vi "SE FP hindbrain ACT.vi"(4 "Manual?":bool=TRUE, 6 "error in":errorcluster, 7 "Act Com":T1, 8 "MHeading":dbl(slide) scale=-45.0..45.0 scale format="%_1f", 9 "MSpeed":dbl(slide) scale=-50.0..50.0 scale format="%#.1g") -> (0 "error out":errorcluster, 1 "Speed":dbl min=-9.0 max=9.0 step=1.0, 2 "Rudder":dbl min=-45.0 max=45.0 step=1.0, 3 "Desired\nSpeed":dbl, 5 "Desired \nRudder":dbl)   [LabVIEW 2014]
doc: "This vi has two functions: it selects between manual and auto mode and it converts the incoming value into speed and rudder control values."
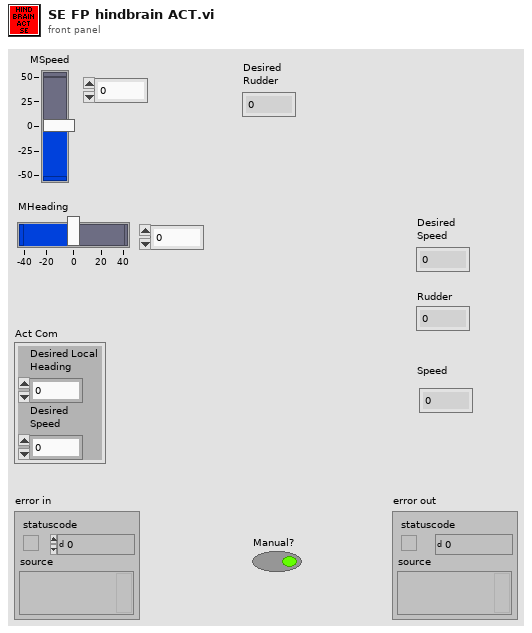
[diagram p1: front panel]
types:
  T1 = cluster{"Desired Local\nHeading":dbl, "Desired\nSpeed":dbl}
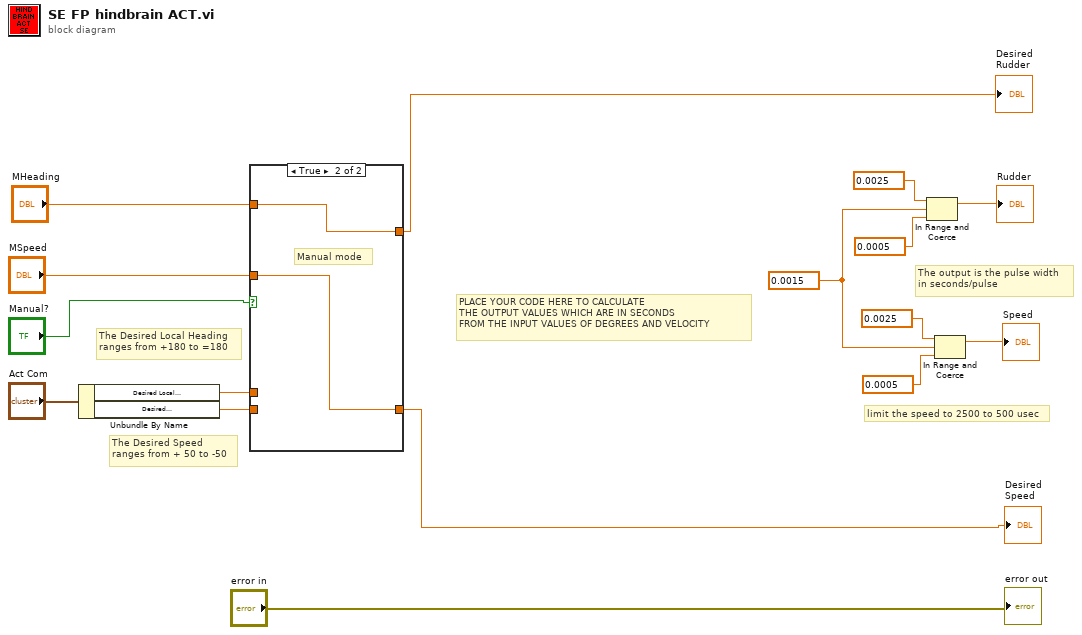
[diagram p0: block diagram]
diagram:
  w3 = 0.0015
  # "PLACE YOUR CODE HERE TO CALCULATE\nTHE OUTPUT VALUES WHICH ARE IN SECONDS\nFROM THE INPUT VALUES OF DEGREES AND VELOCITY"
  # "The output is the pulse width\nin seconds/pulse"
  # "The Desired Local Heading\nranges from +180 to =180"
  # "The Desired Speed\nranges from + 50 to -50"
  # "limit the speed to 2500 to 500 usec"
  n1 = Unbundle By Name("Act Com") -> ("Desired Local\nHeading"=w8:dbl, "Desired\nSpeed"=w7:dbl)
  n2 = case shown="True" "Manual?" {
    tunnel: w8 -> [w18 _]
    tunnel: [w18 w20] -> w2
    tunnel: w7 -> [w17 _]
    tunnel: [w17 w19] -> w1
    tunnel: "MHeading" -> [_ w20]
    tunnel: "MSpeed" -> [_ w19]
    frame False {
      # "Auto mode"
    }
    frame True {
      # "Manual mode"
    }
  }
  "Desired \nRudder" <- w2
  "Desired\nSpeed" <- w1
  n3 = In Range and Coerce(upper limit=0.0025 ("t"), x=w3, lower limit=0.0005 ("t")) -> (coerced(x)=→"Rudder":dbl)  [unwired: 1 out]
  n4 = In Range and Coerce(upper limit=0.0025 ("t"), x=w3, lower limit=0.0005 ("t")) -> (coerced(x)=→"Speed":dbl)  [unwired: 1 out]
  "error out" <- "error in"
